vi "go3Import.vi"(11 "go3 data":path) -> (2 "flows, sccm":dbl[][](array[numeric]), 3 "[o3], ppb":dbl[][](array[numeric]))   [LabVIEW 2011]
uses:
  <vilib>/Utility/file.llb/Read From Spreadsheet File (DBL).vi
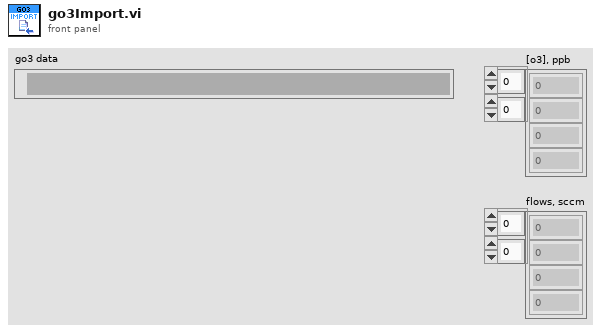
[diagram p1: front panel]
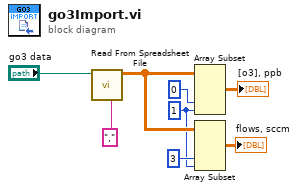
[diagram p0: block diagram]
diagram:
  w5 = 1 ("length")
  n1 = call-poly <vilib>:"Read From Spreadsheet File.vi"("delimiter (\\t)"="," ("delimiter (\\t)"), "file path (dialog if empty)"="go3 data") -> ("all rows"=w7:dbl[][])  [unwired: 5 in, 4 out]
  n2 = Array Subset(array=w7, index (col)=0 ("index"), length (col)=w5) -> (→"[o3], ppb":dbl[][])  [unwired: 2 in]
  n3 = Array Subset(array=w7, index (col)=3 ("index"), length (col)=w5) -> (→"flows, sccm":dbl[][])  [unwired: 2 in]
